vi "Operation.vi"(8 "Error In":errorcluster, 11 "Multiply In":refnum<class "Multiply.lvclass">) -> (0 "Error Out":errorcluster, 2 "C":dbl, 3 "Multiply Out":refnum<class "Multiply.lvclass">)   [LabVIEW 2019, in "Multiply.lvclass"]
uses:
  Multiply.lvclass
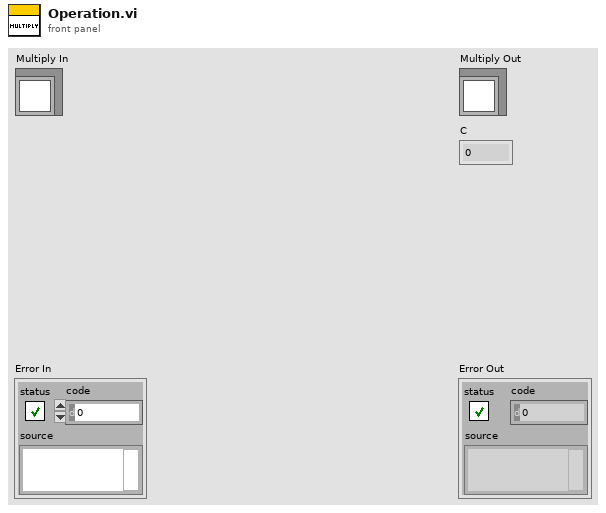
[diagram p1: front panel]
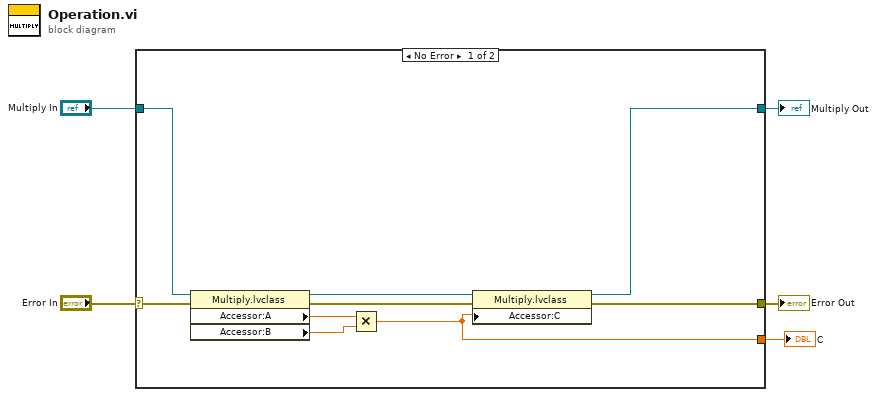
[diagram p0: block diagram]
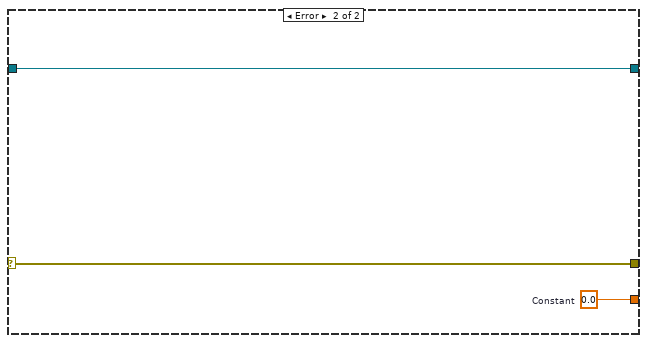
[diagram p2: hidden frame]
diagram:
  n1 = case shown="No Error" "Error In" {
    selector: "Error In" -> [w14 w17]
    tunnel: [w9 w17] -> w4
    tunnel: [w6 w16] -> w2
    tunnel: "Multiply In" -> [w12 w16]
    tunnel: [w7 w15] -> w1
    frame No Error {
      n2 = property class="Multiply.lvclass"(reference=w12, error in=w14) -> (reference out=w8:refnum<class "Multiply.lvclass">, error out=w13:errorcluster, "Accessor:A"=w11:dbl, "Accessor:B"=w10:dbl)
      n3 = Multiply(x=w11, y=w10) -> (x*y=w7:dbl)
      n4 = property class="Multiply.lvclass"(reference=w8, error in=w13, "Accessor:C"=w7) -> (reference out=w6:refnum<class "Multiply.lvclass">, error out=w9:errorcluster)
    }
    frame Error {
      w15 = 0.0  # Constant
    }
  }
  "Error Out" <- w4
  "Multiply Out" <- w2
  "C" <- w1
